vi "Create Writer Endpoint.vi"(6 "writer name":string="//localhost/S4ACS_C1_WRITER", 8 "error in (no error)":errorcluster, 9 "reader name":string="S4GUI_C1_READER", 11 "Stream in":refnum<class "Stream.lvclass">) -> (0 "error out":errorcluster, 3 "Stream out":refnum<class "Stream.lvclass">)   [LabVIEW 2018, in "Stream.lvclass"]
doc: "Create writer endpoint"
uses:
  Stream.lvclass
  Stream.lvclass/Stream.ctl
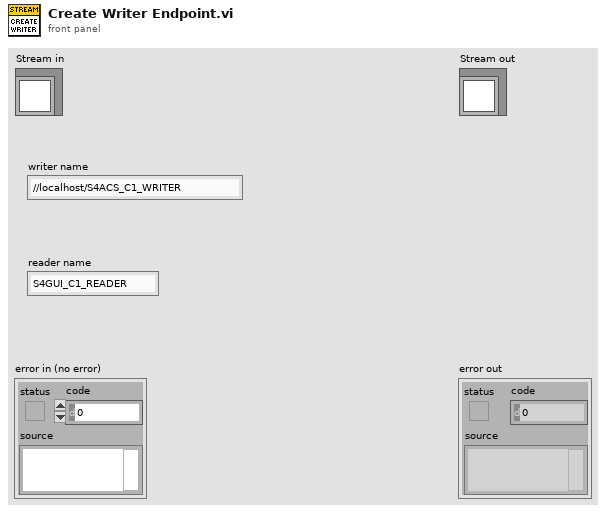
[diagram p1: front panel]
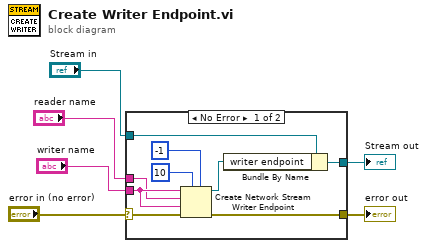
[diagram p0: block diagram]
diagram:
  n1 = case shown="No Error" "error in (no error)" {
    selector: "error in (no error)" -> [w14 w17]
    tunnel: [w15 w17] -> w5
    tunnel: [w11 w16] -> w3
    tunnel: "Stream in" -> [w12 w16]
    tunnel: "reader name" -> [w7 _]
    tunnel: "writer name" -> [w8 _]
    frame No Error {
      n2 = Create Network Stream Writer Endpoint(5:-1 ("timeout in ms (-1)"), 7:10 ("writer buffer size"), 8:w14, 9:w8, 10:w7, 11:w8) -> (0:w15:errorcluster, 3:w9:refnum<k21>)  [unwired: 1 in]
      n3 = Bundle By Name(cluster=w12, "writer endpoint"=w9) -> (w11:refnum<class "Stream.lvclass">)
    }
    frame Error {
    }
  }
  "error out" <- w5
  "Stream out" <- w3
